vi "TouchPanel.AlphanumericGui.vi"(4 "Password Display (F)":bool, 6 "Max Length (70)":i32=70, 8 "Limit to single line (T)":bool=TRUE, 10 "String In":string, 11 "Message In":string) -> (1 "Canceled":bool, 2 "String Out":string)   [LabVIEW 2016]
uses:
  TouchPanel.DriverCommands.ctl
panel:
  in  "Clear":bool
  in  "Shift2":bool
  in  "~\n`":bool
  in  "Tab":bool
  in  "~<\n,":bool
  in  "~?\n/":bool
  in  "~>\n.":bool
  in  "~M\nm":bool
  in  "~N\nn":bool
  in  "~B\nb":bool
  in  "~V\nv":bool
  in  "~C\nc":bool
  in  "~X\nx":bool
  in  "~Z\nz":bool
  in  "~\"\n'":bool
  in  "~:\n;":bool
  in  "~L\nl":bool
  in  "~K\nk":bool
  in  "~J\nj":bool
  in  "~H\nh":bool
  in  "~G\ng":bool
  in  "~F\nf":bool
  in  "~D\nd":bool
  in  "~S\ns":bool
  in  "~A\na":bool
  in  "~}\n]":bool
  in  "~{\n[":bool
  in  "~|\n\\":bool
  in  "~+\n=":bool
  in  "~_\n-":bool
  in  "~P\np":bool
  in  "~O\no":bool
  in  "~I\ni":bool
  in  "~U\nu":bool
  in  "~Y\ny":bool
  in  "~T\nt":bool
  in  "~R\nr":bool
  in  "~E\ne":bool
  in  "~W\nw":bool
  in  "~)\n0":bool
  in  "~(\n9":bool
  in  "~*\n8":bool
  in  "~&\n7":bool
  in  "~^\n6":bool
  in  "~%\n5":bool
  in  "~$\n4":bool
  in  "~#\n3":bool
  in  "~@\n2":bool
  in  "~!\n1":bool
  in  "~Q\nq":bool
  in  "Right":bool
  in  "Left":bool
  out "Message":string
  in  "Insert":bool
  in  "Enter":bool
  in  "CancelButton":bool
  in  "Space":bool
  in  "Shift1":bool
  in  "Capslock":bool
  in  "Text":string
  in  "Backspace":bool
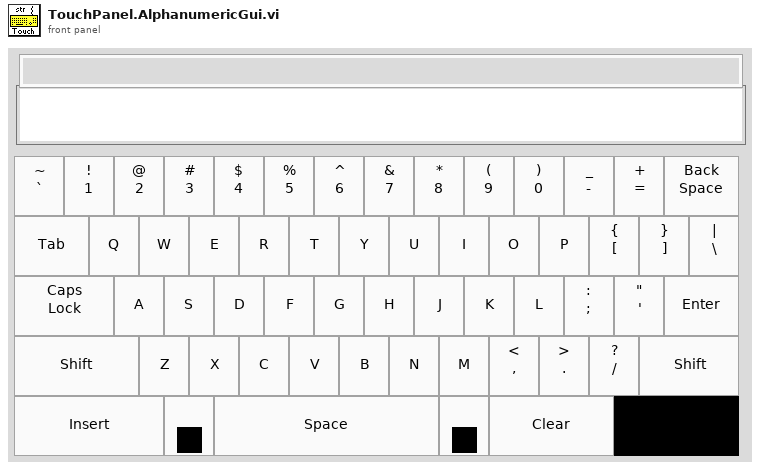
[diagram p1: front panel]
types:
  T1 = typedef "TouchPanel.DriverCommands.ctl" = enum16{"No Command", "Initialize", "Add Character", "Replace Character", "Delete Character", "Move Left", "Move Right", "Update Edit Position"}
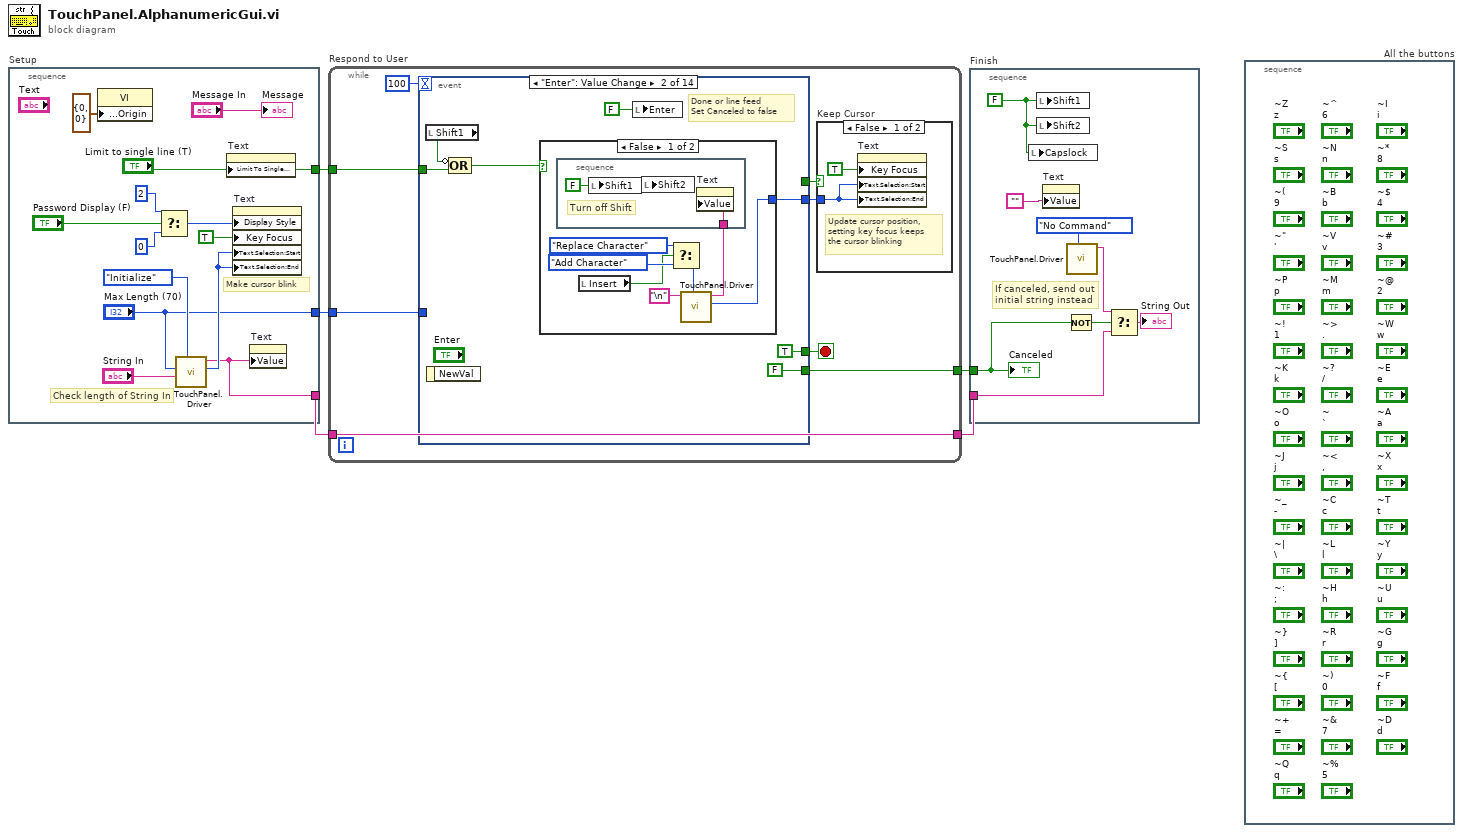
[diagram p0: block diagram]
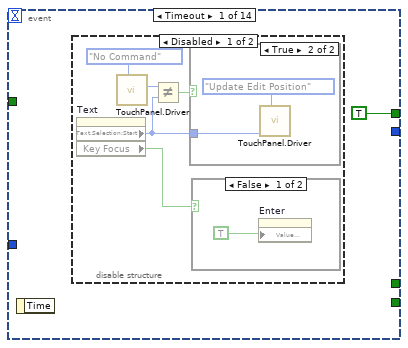
[diagram p3: hidden frame]
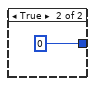
[diagram p7: hidden frame]
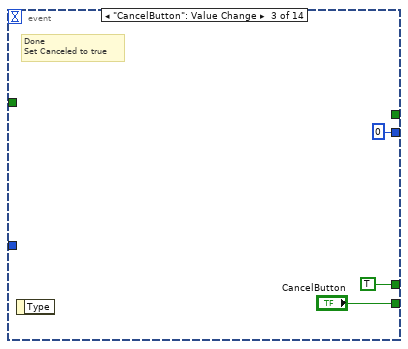
[diagram p8: hidden frame]
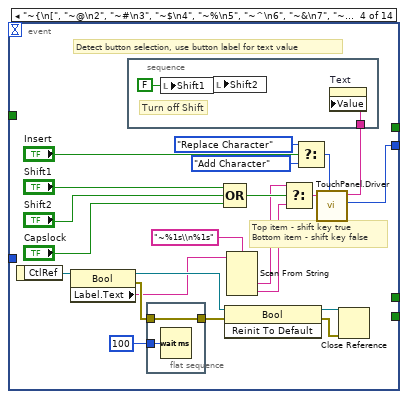
[diagram p9: hidden frame]
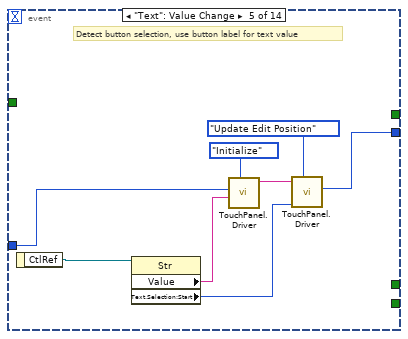
[diagram p10: hidden frame]
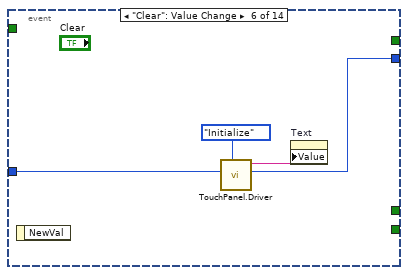
[diagram p11: hidden frame]
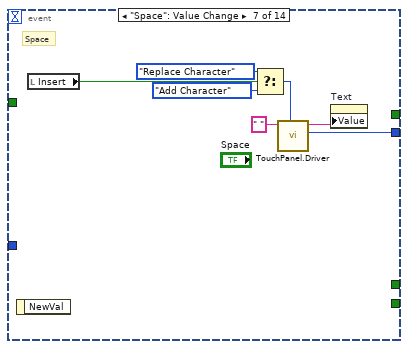
[diagram p12: hidden frame]
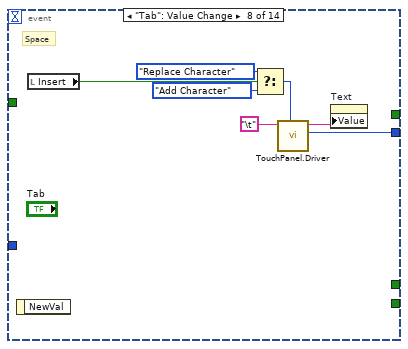
[diagram p13: hidden frame]
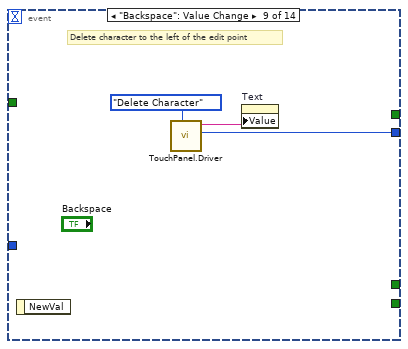
[diagram p14: hidden frame]
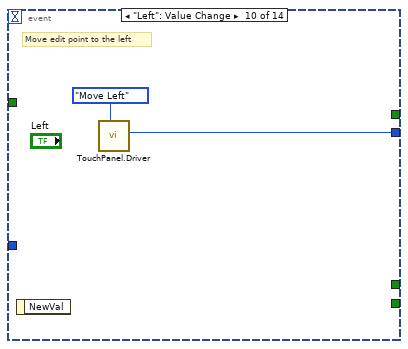
[diagram p15: hidden frame]
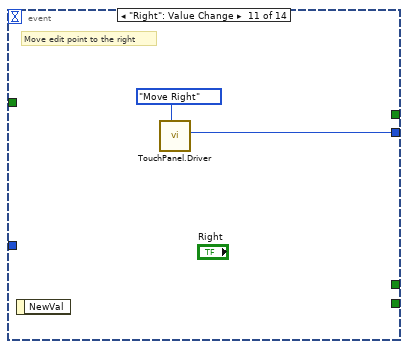
[diagram p16: hidden frame]
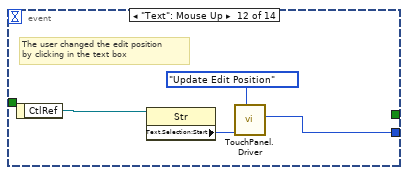
[diagram p17: hidden frame]
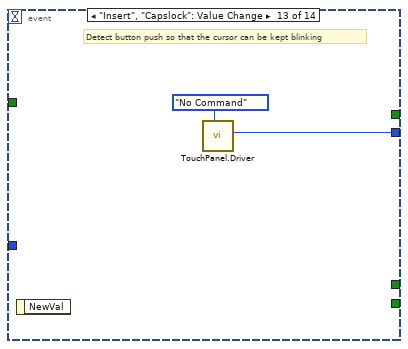
[diagram p18: hidden frame]
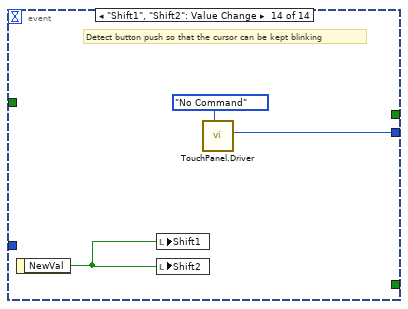
[diagram p19: hidden frame]
diagram:
  n1 = stacked-sequence "Setup" {
    tunnel: [w9] -> w5
    tunnel: ["Max Length (70)"] -> w2
    tunnel: ["Limit to single line (T)"] -> w1
    frame #0 {
      # "Make cursor blink"
      # "Check length of String In"
      n2 = property class="VI"("Front Panel Window:Origin"=cluster{"Horizontal":i16, "Vertical":i16} {"Horizontal"=0, "Vertical"=0}) -> ()  [unwired: 2 in, 2 out]
      n3 = Select(t=u32 2 ("Display Style"), s="Password Display (F)", f=u32 0 ("Display Style")) -> (s? t:f=w14:u32)
      n4 = call "TouchPanel.Driver.vi"("Driver Commands"=TouchPanel.DriverCommands."Initialize", "Initial String"="String In", "Max Length (70)"="Max Length (70)") -> ("Edit Position"=w12:i32, "String Out"=w9:string)  [unwired: 2 in, 5 out]
      n5 = property on="Text" class="Str"("Limit To Single Line?"="Limit to single line (T)") -> ()  [unwired: 2 in, 2 out]
      n6 = property on="Text" class="Str"("Display Style"=w14, "Key Focus"=TRUE, "Text.Selection:Start"=w12, "Text.Selection:End"=w12) -> ()  [unwired: 2 in, 2 out]
      n7 = property on="Text" class="Str"("Value"=w9) -> ()  [unwired: 2 in, 2 out]
      "Message" <- "Message In"
    }
  }
  n8 = while "Respond to User" {
    tunnel: w5 -> [w23]
    tunnel: [w24] -> w4
    tunnel: [w23] -> w3
    tunnel: w2 -> [w22]
    tunnel: w1 -> [w19]
    stop <- w26 stop-if-true
    n9 = event shown="[1] \"Enter\": Value Change" {
      selector: _ -> [_ _ _ _ _ _ _ _ _ _ _ _ _ _]
      dyn-events: _ -> [_ _ _ _ _ _ _ _ _ _ _ _ _ _]
      timeout: 100 -> [_ _ _ _ _ _ _ _ _ _ _ _ _ _]
      tunnel: [_ TRUE TRUE _ _ _ _ _ _ _ _ _ _ _] -> w26
      tunnel: [_ w39 0 ("Edit Position") w71 w85 w92 w98 w106 w111 w114 w115 w117 w121 w124] -> w25
      tunnel: [_ FALSE ("Cancel") "CancelButton" _ _ _ _ _ _ _ _ _ _ _] -> w24
      tunnel: w22 -> [_ _ _ _ w89 w94 _ _ _ _ _ _ _ _]
      tunnel: [TRUE _ _ _ _ _ _ _ _ _ _ _ _ _] -> w20
      tunnel: w19 -> [_ w42 _ _ _ _ _ _ _ _ _ _ _ _]
      event Timeout {
        n10 = event-data() -> ()  [unwired: 2 out]
        n11 = disable-structure shown="Disabled" {
          frame Disabled {
            n12 = property on="Text" class="Str"() -> ("Text.Selection:Start"=w31:u32, "Key Focus"=w30:bool)  [unwired: 2 in, 2 out]
            n13 = call "TouchPanel.Driver.vi"("Driver Commands"=TouchPanel.DriverCommands."No Command") -> ("Edit Position"=w33:i32)  [unwired: 4 in, 6 out]
            n14 = Not Equal?(x=w33, y=w31) -> (x != y?=w32:bool)
            n15 = case shown="True" w32 {
              tunnel: w31 -> [_ w36]
              frame False {
              }
              frame True {
                n16 = call "TouchPanel.Driver.vi"("Driver Commands"=TouchPanel.DriverCommands."Update Edit Position", "New Edit Position"=w36) -> ()  [unwired: 3 in, 7 out]
              }
            }
            n17 = case shown="False" w30 {
              frame False {
                n18 = property on="Enter" class="Bool (strict)"("Value (Signaling)"=TRUE ("Enter")) -> ()  [unwired: 2 in, 2 out]
              }
              frame True {
              }
            }
          }
          frame Enabled {
          }
        }
      }
      event "Enter": Value Change {
        # "Done or line feed\nSet Canceled to false"
        n19 = local read "Shift1"() -> (w41:bool)
        n20 = event-data() -> ()  [unwired: 2 out]
        n21 = Compound Arithmetic op=OR(invert w41, w42) -> (w40:bool)
        n22 = case shown="False" w40 {
          tunnel: [w46 0 ("Edit Position")] -> w39
          frame False {
            n23 = local read "Insert"() -> (w47:bool)
            n24 = Select(t=TouchPanel.DriverCommands."Replace Character" ("Driver Commands"), s=w47, f=TouchPanel.DriverCommands."Add Character" ("Driver Commands")) -> (s? t:f=w49:T1)
            n25 = call "TouchPanel.Driver.vi"("Driver Commands"=w49, "Character"="\n") -> ("Edit Position"=w46:i32, "String Out"=w48:string)  [unwired: 3 in, 5 out]
            n26 = stacked-sequence {
              tunnel: w48 -> [w52]
              frame #0 {
                w53 = FALSE ("Shift")
                # "Turn off Shift"
                n27 = local write "Shift1"(w53) -> ()
                n28 = local write "Shift2"(w53) -> ()
                n29 = property on="Text" class="Str"("Value"=w52) -> ()  [unwired: 2 in, 2 out]
              }
            }
          }
          frame True {
          }
        }
        n30 = local write "Enter"(FALSE ("Enter")) -> ()
      }
      event "CancelButton": Value Change {
        # "Done\nSet Canceled to true"
        n31 = event-data() -> ()  [unwired: 2 out]
      }
      event "~{\n[", "~@\n2", "~#\n3", "~$\n4", "~%\n5", "~^\n6", "~&\n7", "~*\n8", "~(\n9", "~)\n0", "~_\n-", "~+\n=", "~|\n\\", "~Q\nq", "~W\nw", "~E\ne", "~R\nr", "~T\nt", "~Y\ny", "~U\nu", "~I\ni", "~O\no", "~P\np", "~A\na", "~S\ns", "~D\nd", "~F\nf", "~G\ng", "~H\nh", "~J\nj", "~K\nk", "~L\nl", "~:\n;", "~\"\n'", "~Z\nz", "~X\nx", "~C\nc", "~V\nv", "~B\nb", "~N\nn", "~M\nm", "~<\n,", "~>\n.", "~?\n/", "~}\n]", "~!\n1", "~\n`": Value Change {
        # "Top item - shift key true\nBottom item - shift key false"
        # "Detect button selection, use button label for text value"
        n32 = event-data() -> ("CtlRef"=w65:refnum<vi>)  [unwired: 1 out]
        n33 = property class="Bool"(reference=w65) -> (reference out=w62:refnum<vi>, error out=w61:errorcluster, "Label.Text"=w58:string)  [unwired: 1 in]
        n34 = flat-sequence {
          tunnel: [w81] -> w60
          tunnel: w61 -> [w81]
          tunnel: u32 100 ("milliseconds to wait") -> [w80]
          frame #0 {
            n35 = Wait (ms)(milliseconds to wait=w80) -> ()  [unwired: 1 out]
          }
        }
        n36 = Compound Arithmetic op=OR("Shift1", "Shift2", "Capslock") -> (w78:bool)
        n37 = invoke class="Bool" method="Reinit To Default"(reference=w62, error in=w60) -> (reference out=w64:refnum<vi>, error out=w63:errorcluster)  [unwired: 1 in, 1 out]
        n38 = Scan From String(format string="~%1s\\n%1s", input string=w58) -> (output 1=w77:string, output 2=w76:string)  [unwired: 2 in, 5 out]
        n39 = Select(t=w77, s=w78, f=w76) -> (s? t:f=w75:string)
        n40 = Select(t=TouchPanel.DriverCommands."Replace Character" ("Driver Commands"), s="Insert", f=TouchPanel.DriverCommands."Add Character" ("Driver Commands")) -> (s? t:f=w74:T1)
        n41 = call "TouchPanel.Driver.vi"("Driver Commands"=w74, "Character"=w75) -> ("Edit Position"=w71:i32, "String Out"=w67:string)  [unwired: 3 in, 5 out]
        n42 = stacked-sequence {
          tunnel: w67 -> [w82]
          frame #0 {
            w83 = FALSE ("Shift")
            # "Turn off Shift"
            n43 = local write "Shift1"(w83) -> ()
            n44 = local write "Shift2"(w83) -> ()
            n45 = property on="Text" class="Str"("Value"=w82) -> ()  [unwired: 2 in, 2 out]
          }
        }
        n46 = Close Reference(reference=w64, error in (no error)=w63) -> ()  [unwired: 1 out]
      }
      event "Text": Value Change {
        # "Detect button selection, use button label for text value"
        n47 = event-data() -> ("CtlRef"=w91:refnum<vi>)  [unwired: 1 out]
        n48 = property class="Str"(reference=w91) -> ("Value"=w84:string, "Text.Selection:Start"=w86:u32)  [unwired: 1 in, 2 out]
        n49 = call "TouchPanel.Driver.vi"("Driver Commands"=TouchPanel.DriverCommands."Initialize", "Initial String"=w84, "Max Length (70)"=w89) -> ("String Out"=w88:string)  [unwired: 2 in, 6 out]
        n50 = call "TouchPanel.Driver.vi"("Driver Commands"=TouchPanel.DriverCommands."Update Edit Position", "New Edit Position"=w86, "Character"=w88) -> ("Edit Position"=w85:i32)  [unwired: 2 in, 6 out]
      }
      event "Clear": Value Change {
        n51 = event-data() -> ()  [unwired: 2 out]
        n52 = call "TouchPanel.Driver.vi"("Driver Commands"=TouchPanel.DriverCommands."Initialize", "Max Length (70)"=w94) -> ("Edit Position"=w92:i32, "String Out"=w93:string)  [unwired: 3 in, 5 out]
        n53 = property on="Text" class="Str"("Value"=w93) -> ()  [unwired: 2 in, 2 out]
      }
      event "Space": Value Change {
        # "Space"
        n54 = event-data() -> ()  [unwired: 2 out]
        n55 = local read "Insert"() -> (w97:bool)
        n56 = Select(t=TouchPanel.DriverCommands."Replace Character" ("Driver Commands"), s=w97, f=TouchPanel.DriverCommands."Add Character" ("Driver Commands")) -> (s? t:f=w99:T1)
        n57 = call "TouchPanel.Driver.vi"("Driver Commands"=w99, "Character"=" ") -> ("Edit Position"=w98:i32, "String Out"=w96:string)  [unwired: 3 in, 5 out]
        n58 = property on="Text" class="Str"("Value"=w96) -> ()  [unwired: 2 in, 2 out]
      }
      event "Tab": Value Change {
        # "Space"
        n59 = event-data() -> ()  [unwired: 2 out]
        n60 = local read "Insert"() -> (w105:bool)
        n61 = Select(t=TouchPanel.DriverCommands."Replace Character" ("Driver Commands"), s=w105, f=TouchPanel.DriverCommands."Add Character" ("Driver Commands")) -> (s? t:f=w107:T1)
        n62 = call "TouchPanel.Driver.vi"("Driver Commands"=w107, "Character"="\t") -> ("Edit Position"=w106:i32, "String Out"=w104:string)  [unwired: 3 in, 5 out]
        n63 = property on="Text" class="Str"("Value"=w104) -> ()  [unwired: 2 in, 2 out]
      }
      event "Backspace": Value Change {
        # "Delete character to the left of the edit point"
        n64 = event-data() -> ()  [unwired: 2 out]
        n65 = call "TouchPanel.Driver.vi"("Driver Commands"=TouchPanel.DriverCommands."Delete Character") -> ("Edit Position"=w111:i32, "String Out"=w110:string)  [unwired: 4 in, 5 out]
        n66 = property on="Text" class="Str"("Value"=w110) -> ()  [unwired: 2 in, 2 out]
      }
      event "Left": Value Change {
        # "Move edit point to the left"
        n67 = event-data() -> ()  [unwired: 2 out]
        n68 = call "TouchPanel.Driver.vi"("Driver Commands"=TouchPanel.DriverCommands."Move Left") -> ("Edit Position"=w114:i32)  [unwired: 4 in, 6 out]
      }
      event "Right": Value Change {
        # "Move edit point to the right"
        n69 = event-data() -> ()  [unwired: 2 out]
        n70 = call "TouchPanel.Driver.vi"("Driver Commands"=TouchPanel.DriverCommands."Move Right") -> ("Edit Position"=w115:i32)  [unwired: 4 in, 6 out]
      }
      event "Text": Mouse Up {
        # "The user changed the edit position\nby clicking in the text box"
        n71 = event-data() -> ("CtlRef"=w120:refnum<vi>)  [unwired: 1 out]
        n72 = property class="Str"(reference=w120) -> ("Text.Selection:Start"=w119:u32)  [unwired: 1 in, 2 out]
        n73 = call "TouchPanel.Driver.vi"("Driver Commands"=TouchPanel.DriverCommands."Update Edit Position", "New Edit Position"=w119) -> ("Edit Position"=w117:i32)  [unwired: 3 in, 6 out]
      }
      event "Insert", "Capslock": Value Change {
        # "Detect button push so that the cursor can be kept blinking"
        n74 = event-data() -> ()  [unwired: 2 out]
        n75 = call "TouchPanel.Driver.vi"("Driver Commands"=TouchPanel.DriverCommands."No Command") -> ("Edit Position"=w121:i32)  [unwired: 4 in, 6 out]
      }
      event "Shift1", "Shift2": Value Change {
        # "Detect button push so that the cursor can be kept blinking"
        n76 = event-data() -> ("NewVal"=w123:bool)  [unwired: 1 out]
        n77 = local write "Shift1"(w123) -> ()
        n78 = local write "Shift2"(w123) -> ()
        n79 = call "TouchPanel.Driver.vi"("Driver Commands"=TouchPanel.DriverCommands."No Command") -> ("Edit Position"=w124:i32)  [unwired: 4 in, 6 out]
      }
    }
    n80 = case "Keep Cursor" shown="False" w20 {
      tunnel: w25 -> [w27 _]
      frame False {
        # "Update cursor position,\nsetting key focus keeps\nthe cursor blinking"
        n81 = property on="Text" class="Str"("Key Focus"=TRUE, "Text.Selection:Start"=w27, "Text.Selection:End"=w27) -> ()  [unwired: 2 in, 2 out]
      }
      frame True {
      }
    }
  }
  n82 = stacked-sequence "Finish" {
    tunnel: w4 -> [w132]
    tunnel: w3 -> [w129]
    frame #0 {
      w126 = FALSE ("Shift1")
      # "If canceled, send out\ninitial string instead"
      n83 = local write "Capslock"(w126) -> ()
      n84 = local write "Shift1"(w126) -> ()
      n85 = local write "Shift2"(w126) -> ()
      n86 = property on="Text" class="Str"("Value"="") -> ()  [unwired: 2 in, 2 out]
      n87 = Not(x=w132) -> (.not. x?=w130:bool)
      n88 = call "TouchPanel.Driver.vi"("Driver Commands"=TouchPanel.DriverCommands."No Command") -> ("String Out"=w128:string)  [unwired: 4 in, 6 out]
      n89 = Select(t=w128, s=w130, f=w129) -> (s? t:f=→"String Out":string)
      "Canceled" <- w132
    }
  }
  n90 = stacked-sequence "All the buttons" {
    frame #0 {
    }
  }
